vi "Control Relay (boolean).vi"(8 "error in (no error)":errorcluster, 9 "Array":bool[](array[boolean])) -> (0 "error out":errorcluster)   [LabVIEW 2019, in "Relay-Box.lvclass"]
uses:
  <userlib>/LevyLab/Relay Box/Relay-Box.lvclass
  <userlib>/LevyLab/Relay Box/Relay-Box.lvclass/Relay-Box.ctl
  <userlib>/LevyLab/Relay Box/D2XX_Functions/D2XX_Functions.lvlib
panel:
  out "FT_Status out":u32(ring) items=["FT_OK", "FT_INVALID_HANDLE", "FT_DEVICE_NOT_FOUND", "FT_DEVICE_NOT_OPENED", "FT_IO_ERROR", "FT_INSUFFICIENT_RESOURCES", "FT_INVALID_PARAMETER", "FT_INVALID_BAUD_RATE", "FT_DEVICE_NOT_OPENED_FOR_ERASE", "FT_DEVICE_NOT_OPENED_FOR_WRITE", "FT_FAILED_TO_WRITE_DEVICE", "FT_EEPROM_READ_FAILED", "FT_EEPROM_WRITE_FAILED", "FT_EEPROM_ERASE_FAILED", "FT_EEPROM_NOT_PRESENT", "FT_EEPROM_NOT_PROGRAMMED", "FT_INVALID_ARGS", "FT_NOT_SUPPORTED", "FT_OTHER_ERROR"]
  # "Discharge tip"
  # "0 ohm"
  # "100k ohm"
  # "10M ohm"
  # "1Gohm"
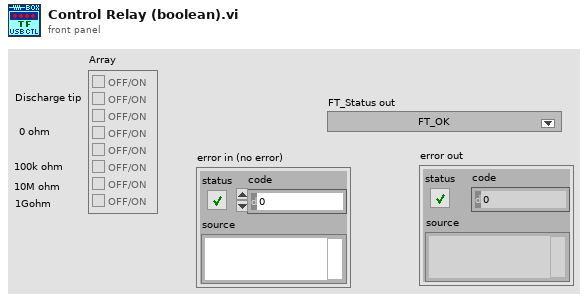
[diagram p1: front panel]
types:
  T1 = cluster{"Signature 1":u32, "Signature 2":u32, "Version":u32, "Vendor ID":u16, "Product ID":u16, "Manufacturer":string, "Manufacturer ID":string, "Description":string, "Serial Number":string, "Max Power (mA)":u16, "PnP":u16, "Self Powered":u16, "Remote Wake-Up":u16, "Rev4":u8, "Iso In":u8, "Iso Out":u8, "Pull Down Enable":u8, "Serial Number Enable":u8, "USB Version Enable":u8, "USB Version":u16, "Rev5":u8, "Iso In A":u8, "Iso In B":u8, "Iso Out A":u8, "Iso Out B":u8, "Pull Down Enable 5":u8, "Serial Number Enable 5":u8, "USB Version Enable 5":u8, "USB Version 5":u16, "A Is High Current":u8, "B Is High Current":u8, "A Is 245 FIFO":u8, "A Is CPU FIFO":u8, "A Is Fast Serial":u8, "A Is VCP":u8, "B Is 245 FIFO":u8, "B Is CPU FIFO":u8, "B Is Fast Serial":u8, "B Is VCP":u8, "Use Ext Osc":u8, "High Drive IOs":u8, "Endpoint Size":u8, "Pull Down Enable R":u8, "Serial Number Enable R":u8, "Invert TXD":u8, "Invert RXD":u8, "Invert RTS":u8, "Invert CTS":u8, "Invert DTR":u8, "Invert DSR":u8, "Invert DCD":u8, "Invert RI":u8, "CBus0":u8, "CBus1":u8, "CBus2":u8, "CBus3":u8, "CBus4":u8, "R Is VCP":u8, "Pull Down Enable 7":u8, "Serial Number Enable 7":u8, "AL Slow Slew":u8, "AL Schmitt Input":u8, "AL Drive Current":u8, "AH Slow Slew":u8, "AH Schmitt Input":u8, "AH Drive Current":u8, "BL Slow Slew":u8, "BL Schmitt Input":u8, "BL Drive Current":u8, "BH Slow Slew":u8, "BH Schmitt Input":u8, "BH Drive Current":u8, "A Is 245 FIFO 7":u8, "A Is CPU FIFO 7":u8, "A Is Fast Serial 7":u8, "A Is VCP 7":u8, "B Is 245 FIFO 7":u8, "B Is CPU FIFO 7":u8, "B Is Fast Serial 7":u8, "B Is VCP 7":u8, "PowerSaveEnable":u8, "Pull Down Enable 8":u8, "Serial Number Enable 8":u8, "A Slow Slew":u8, "A Schmitt Input":u8, "A Drive Current":u8, "B Slow Slew":u8, "B Schmitt Input":u8, "B Drive Current":u8, "C Slow Slew":u8, "C Schmitt Input":u8, "C Drive Current":u8, "D Slow Slew":u8, "D Schmitt Input":u8, "D Drive Current":u8, "A RI Is TXDEN":u8, "B RI Is TXDEN":u8, "C RI Is TXDEN":u8, "D RI Is TXDEN":u8, "A Is VCP 8":u8, "B Is VCP 8":u8, "C Is VCP 8":u8, "D Is VCP 8":u8}
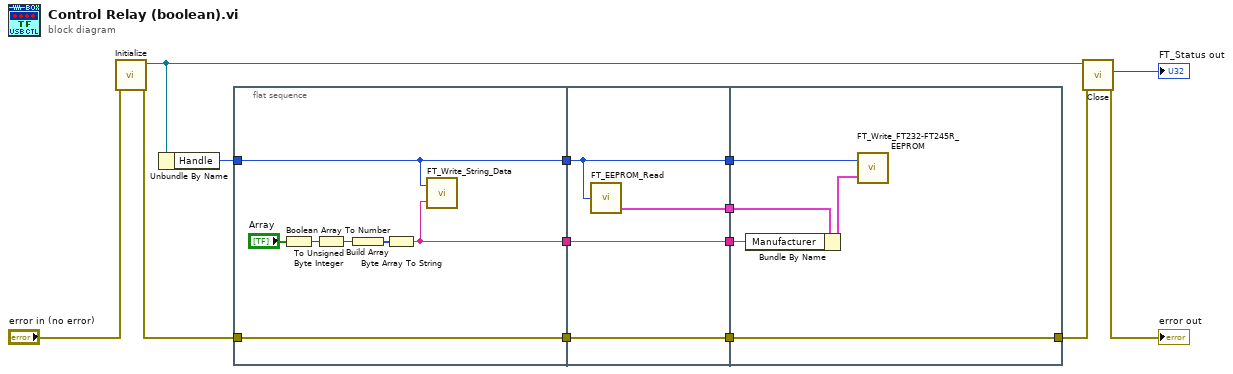
[diagram p0: block diagram]
diagram:
  n1 = call <userlib>:"Initialize.vi"("error in (no error)"="error in (no error)") -> ("error out"=w5:errorcluster, "Relay-Box out"=w4:refnum<class "Relay-Box.lvclass">)  [unwired: 9 in]
  n2 = Unbundle By Name(w4) -> ("Handle"=w1:u32)
  n3 = flat-sequence {
    tunnel: [w16] -> w14
    tunnel: [w21] -> w13
    tunnel: [w15] -> w12
    tunnel: w5 -> [w21]
    tunnel: w1 -> [w16]
    tunnel: w14 -> [w24]
    tunnel: [w24] -> w11
    tunnel: w13 -> [w25]
    tunnel: [w25] -> w10
    tunnel: [w22] -> w9
    tunnel: [w23] -> w8
    tunnel: w12 -> [w23]
    tunnel: w11 -> [w26]
    tunnel: w10 -> [w30]
    tunnel: w9 -> [w28]
    tunnel: w8 -> [w29]
    tunnel: [w30] -> w2
    frame #0 {
      n4 = Boolean Array To Number(Boolean array="Array") -> (number=w18:u32)
      n5 = To Unsigned Byte Integer(number=w18) -> (unsigned 8bit integer=w20:u8)
      n6 = Build Array(w20) -> (w19:u8[])
      n7 = Byte Array To String(unsigned byte array=w19) -> (string=w15:string)
      n8 = call <userlib>:"FT_Write_String_Data.vi"("Buffer"=w15, "Handle"=w16) -> ()  [unwired: 2 out]
    }
    frame #1 {
      n9 = call <userlib>:"FT_EEPROM_Read.vi"("Handle"=w24) -> ("output cluster"=w22:T1)  [unwired: 2 out]
    }
    frame #2 {
      n10 = Bundle By Name(cluster=w28, "Manufacturer"=w29) -> (w27:T1)
      n11 = call <userlib>:"FT_Write_FT232-FT245R_EEPROM.vi"("FT232-FT245R EEPROM Contents"=w27, "Handle"=w26) -> ()  [unwired: 1 out]
    }
  }
  n12 = call <userlib>:"Close.vi"("error in (no error)"=w2, "Relay-Box in"=w4) -> ("error out"=→"error out":errorcluster, "FT_Status"=→"FT_Status out":u32)  [unwired: 7 in, 1 out]
